vi "Compare Calls.vi"(8 "error in (no error)":errorcluster, 9 "VI Call 2":refnum<class "VI Call.lvclass">, 10 "VI Call 1":refnum<class "VI Call.lvclass">, 11 "String Argument Matching Comparator in":refnum<class "String Argument Matching Comparator.lvclass">) -> (0 "error out":errorcluster, 1 "Description":string, 2 "Equal?":bool)   [LabVIEW 2020, in "String Argument Matching Comparator.lvclass"]
uses:
  String Argument Matching Comparator.lvclass
  Framework/VI Call/VI Call.lvclass
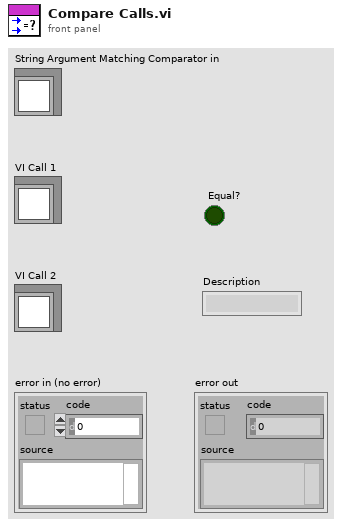
[diagram p1: front panel]
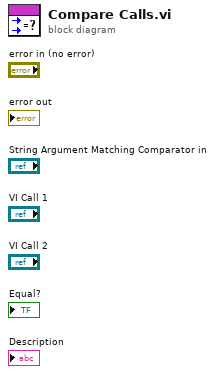
[diagram p0: block diagram]
diagram:
